vi "Send Data Statistics to Notebook.vi"(6 "Data Axis (Y: F)":bool, 7 "Graph Caption":string, 8 "Error In":errorcluster, 9 "Bin":dbl, 10 "Data Statistics":T1, 11 "Plot Name":string) -> (0 "Error Out":errorcluster)   [LabVIEW 2019]
uses:
  Data Statistics.ctl
  Notebook/Notebook.lvlib
  Histogram Window.lvlib
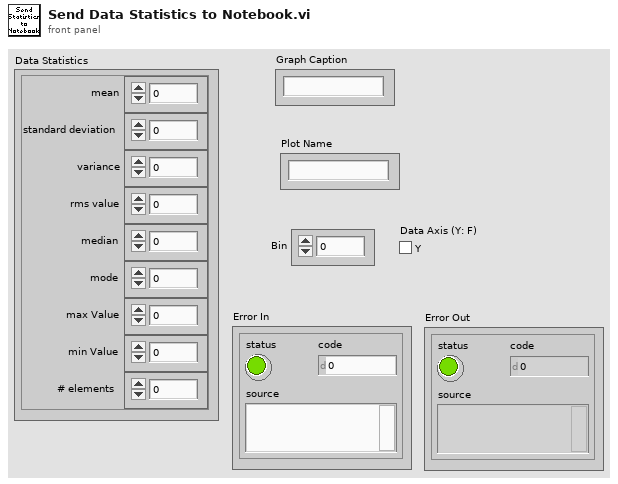
[diagram p1: front panel]
types:
  T1 = typedef "Histogram Window.lvlib/Data Statistics.ctl" = cluster{"mean":dbl, "standard deviation":dbl, "variance":dbl, "rms value":dbl, "median":dbl, "mode":dbl, "max Value":dbl, "min Value":dbl, "# elements  ":dbl}
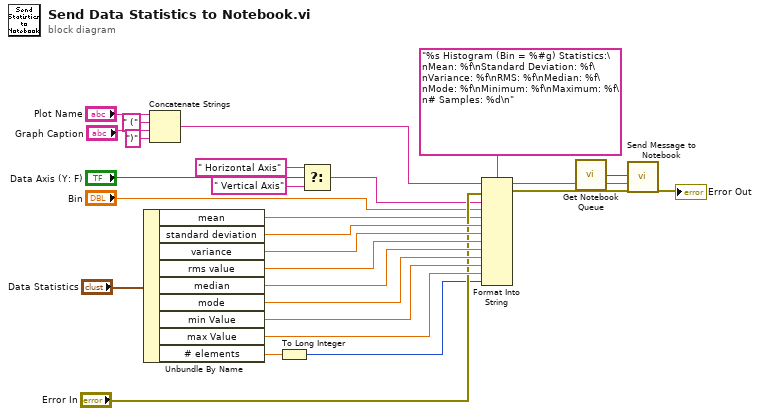
[diagram p0: block diagram]
diagram:
  n1 = Unbundle By Name("Data Statistics") -> ("mean"=w7:dbl, "standard deviation"=w24:dbl, "variance"=w23:dbl, "rms value"=w22:dbl, "median"=w21:dbl, "mode"=w20:dbl, "min Value"=w19:dbl, "max Value"=w18:dbl, "# elements"=w17:dbl)
  n2 = Concatenate Strings("Plot Name", " (" ("string"), "Graph Caption", ")" ("string")) -> (w4:string)
  n3 = To Long Integer(number=w17) -> (32bit integer=w8:i32)
  n4 = Select(t=" Horizontal Axis", s="Data Axis (Y: F)", f=" Vertical Axis") -> (s? t:f=w3:string)
  n5 = Format Into String(format string="%s Histogram (Bin = %#g) Statistics:\nMean: %f\nStandard Deviation: %f\nVariance: %f\nRMS: %f\nMedian: %f\nMode: %f\nMinimum: %f\nMaximum: %f\n# Samples: %d\n", initial string=w4, error in="Error In", w3, "Bin", w7, w24, w23, w22, w21, w20, w19, w18, w8) -> (resulting string=w16:string, error out=w15:errorcluster)
  n6 = call "Get Notebook Queue.vi"() -> ("Notebook Queue"=w13:refnum<queue>)  [unwired: 9 in]
  n7 = call "Send Message to Notebook.vi"("Notebook Queue"=w13, "Message"=w16, "Error In"=w15) -> ("Error Out"=→"Error Out":errorcluster)  [unwired: 16 in]
